vi "Connect.vi"(8 "error in (no error)":errorcluster, 11 "DataReceiver in":refnum<class "DataReceiver.lvclass">) -> (0 "error out":errorcluster, 3 "DataReceiver out":refnum<class "DataReceiver.lvclass">)   [LabVIEW 2010, in "DataReceiver.lvclass"]
uses:
  DataReceiver.lvclass
  DataReceiver.lvclass/DataReceiver.ctl
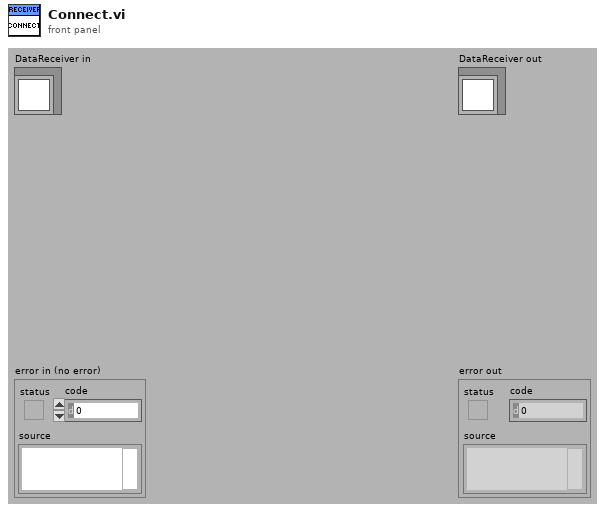
[diagram p1: front panel]
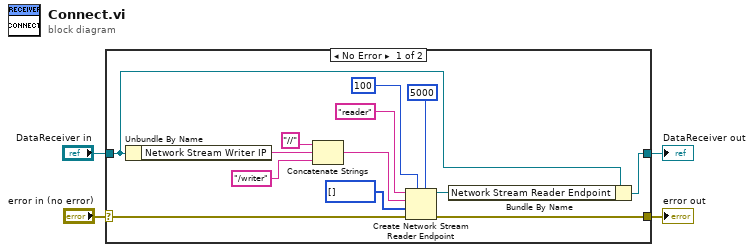
[diagram p0: block diagram]
diagram:
  n1 = case shown="No Error" "error in (no error)" {
    selector: "error in (no error)" -> [w10 w19]
    tunnel: [w9 w19] -> w3
    tunnel: [w7 w18] -> w1
    tunnel: "DataReceiver in" -> [w8 w18]
    frame No Error {
      n2 = Unbundle By Name(w8) -> ("Network Stream Writer IP"=w11:string)
      n3 = Concatenate Strings("//" ("reader url"), w11, "/writer" ("string")) -> (w12:string)
      n4 = Create Network Stream Reader Endpoint(5:5000 ("timeout in ms (-1)"), 7:100 ("reader buffer size"), 8:w10, 9:i32[] [], 10:w12, 11:"reader" ("writer name")) -> (0:w9:errorcluster, 3:w6:refnum<k21>)
      n5 = Bundle By Name(cluster=w8, "Network Stream Reader Endpoint"=w6) -> (w7:refnum<class "DataReceiver.lvclass">)
    }
    frame Error {
    }
  }
  "error out" <- w3
  "DataReceiver out" <- w1
